vi "DISP_WIND_ANN_TRAC_STAT.vi"(0 "VISA IN":refnum<visa-resource-name>, 1 "ON |OFF":bool, 5 "error in":errorcluster, 7 "Window":i32) -> (14 "VISA Out":refnum<visa-resource-name>, 19 "error out":errorcluster)   [LabVIEW 2018, in "PNA-X.lvlib"]
doc: "DISPlay:WINDow<wnum>:ANNotation:TRACe:STATe <ON | OFF> \n(Read-Write) Specifies whether to show or hide the Trace Status buttons on the left of the display. \nParameters \n<wnum> Any existing window number. If unspecified, value is set to 1. \n<ON | OFF> ON (or 1) - turns the buttons ON. \nOFF (or 0) - turns the buttons OFF. \nExamples DISP:WIND:ANN:TRAC:STAT ON \ndisplay:window:annotation:trace:state off \nQuery Syntax DISPlay:WINDow:ANNotation:TRACe:STATe? \nReturn Type Boolean (1 = ON, 0 = OFF) \nDefault ON"
uses:
  PNA-X.lvlib
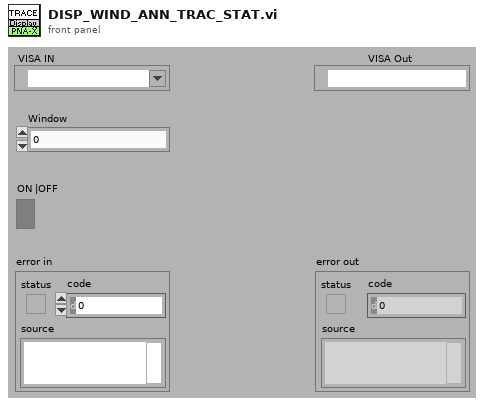
[diagram p1: front panel]
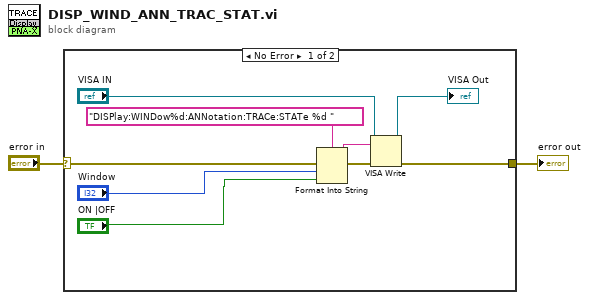
[diagram p0: block diagram]
diagram:
  n1 = case shown="No Error" "error in" {
    selector: "error in" -> [w11 w12]
    tunnel: [w6 w12] -> w1
    frame No Error {
      n2 = Format Into String(format string="DISPlay:WINDow%d:ANNotation:TRACe:STATe %d " ("Cmdline"), error in=w11, "Window", "ON |OFF") -> (resulting string=w9:string, error out=w10:errorcluster)  [unwired: 1 in]
      n3 = VISA Write(VISA resource name="VISA IN", write buffer=w9, error in (no error)=w10) -> (VISA resource name out=→"VISA Out":refnum<visa-resource-name>, error out=w6:errorcluster)  [unwired: 1 out]
    }
    frame Error {
    }
  }
  "error out" <- w1
